vi "Initialize and Configure (No Objects).vi"(6 "trigger mode (0:internal)":u16(ring) items=["internal - continuous trigger", "external - rear panel trigger with delay", "external - bus trigger with delay", "external - rear panel trigger", "external - bus trigger"], 7 "function (0:volts DC)":u16(ring) items=["volts DC", "volts AC", "2-wire k.ohms", "4-wire k.ohms", "mA DC", "mA AC"], 8 "error in (no error)":errorcluster, 9 "rate (0:slow)":u16(ring) items=["slow", "medium", "fast"], 10 "range (0:auto)":u16(ring) items=["autorange", "200mV, 200 ohms", "2V, 2 kohms", "20V, 20 kohms", "200V, 200 kohms", "1000Vdc, 700 Vac, 2 Mohms", "20 Mohms", "20 mV, 20 ohms"], 11 "input cluster":T1) -> (0 "error out":errorcluster, 3 "output cluster":T1)   [LabVIEW 2009]
doc: "Initializes and configures the Fluke Multimeter."
uses:
  Global/GPIB Numbers.vi
  Fluke 8840/Fluke 8840.lvlib
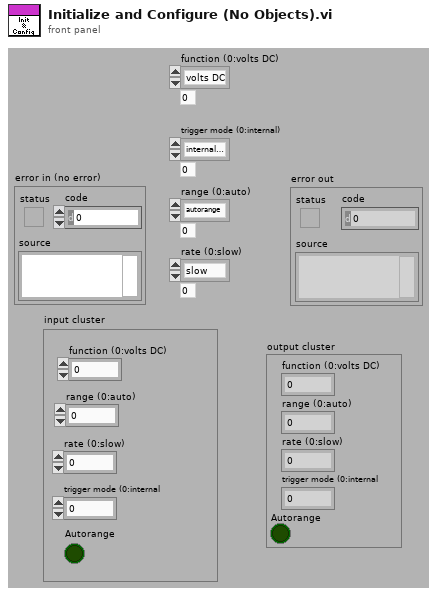
[diagram p1: front panel]
types:
  T1 = cluster{"function (0:volts DC)":i16, "range (0:auto)":i16, "rate (0:slow)":i16, "trigger mode (0:internal":i16, "Autorange":bool}
  T2 = typedef "GPIB Type Def.ctl" = cluster{"Name":string, "bus":dbl, "GPIB":dbl, "GPIB as string":string, "byte":i32, "VISA Resource Name":refnum<visa-resource-name>}
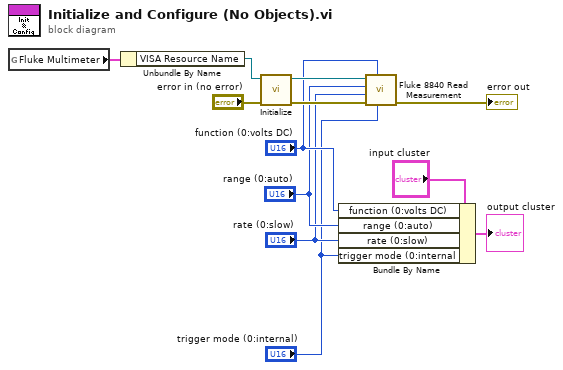
[diagram p0: block diagram]
diagram:
  n1 = global read "GPIB Numbers.vi" "Fluke Multimeter"() -> (w5:T2)
  n2 = Unbundle By Name(w5) -> ("VISA Resource Name"=w2:refnum<visa-resource-name>)
  n3 = call "Initialize.vi"("error in (no error)"="error in (no error)", "VISA resource name"=w2) -> ("error out"=w11:errorcluster, "VISA resource name out"=w12:refnum<visa-resource-name>)  [unwired: 8 in]
  n4 = Bundle By Name(cluster="input cluster", "function (0:volts DC)"="function (0:volts DC)", "range (0:auto)"="range (0:auto)", "rate (0:slow)"="rate (0:slow)", "trigger mode (0:internal"="trigger mode (0:internal)") -> (→"output cluster":T1)
  n5 = call "Fluke 8840 Read Measurement.vi"("trigger mode (0:internal)"="trigger mode (0:internal)", "function (0:volts DC)"="function (0:volts DC)", "error in (no error)"=w11, "rate (0:slow)"="rate (0:slow)", "range (0:auto)"="range (0:auto)", "VISA resource name"=w12) -> ("error out"=→"error out":errorcluster)  [unwired: 2 in, 3 out]
